vi "OUTPUT_DATA_PACKING_TYPE - Type.vi"(8 "error in (no error)":errorcluster) -> (0 "error out":errorcluster, 3 "OUTPUT_DATA_PACKING_TYPE_VALUE":i32)   [LabVIEW 2013]
doc: "<b>Buffer policy settings can be only unsafe in xiAPI LabVIEW library</b>\nUNSAFE : User gets pointer to internally allocated circle buffer and data may be overwritten by device.\nSAFE : Data from device will be copied to user allocated buffer or xiApi allocated memory."
uses:
  OUTPUT_DATA_PACKING_TYPE.ctl
  C:/Projects/Cameras3.x/xiLib/xiLIB_64bit/xiLIB/xiCamLib/API/x64/xiApi.NETX64.dll
  xiLIB_64bit/xiLIB/xiCamLib/API/x64/xiApi.NETX64.dll
panel:
  in  "OUTPUT_DATA_PACKING_TYPE":T1
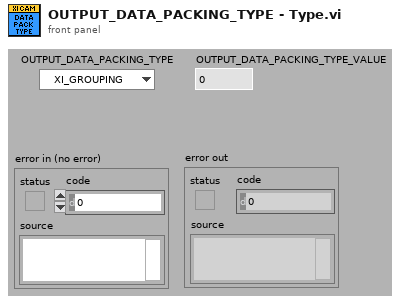
[diagram p1: front panel]
types:
  T1 = typedef "OUTPUT_DATA_PACKING_TYPE.ctl" = enum16{"XI_GROUPING", "PFNC_LSB_PACKING"}
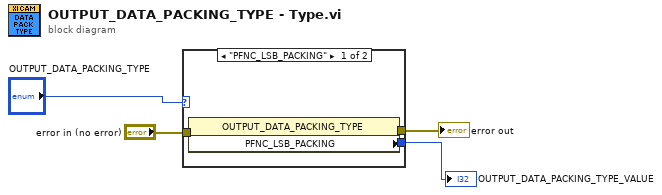
[diagram p0: block diagram]
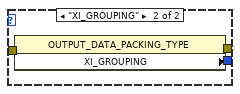
[diagram p2: hidden frame]
diagram:
  n1 = case shown="\"PFNC_LSB_PACKING\"" "OUTPUT_DATA_PACKING_TYPE" {
    tunnel: "error in (no error)" -> [w7 w10]
    tunnel: [w6 w9] -> w3
    tunnel: [w5 w8] -> w2
    frame "PFNC_LSB_PACKING" {
      n2 = property class="OUTPUT_DATA_PACKING_TYPE"(error in=w7) -> (error out=w6:errorcluster, "PFNC_LSB_PACKING"=w5:i32)  [unwired: 1 in, 1 out]
    }
    frame "XI_GROUPING" {
      n3 = property class="OUTPUT_DATA_PACKING_TYPE"(error in=w10) -> (error out=w9:errorcluster, "XI_GROUPING"=w8:i32)  [unwired: 1 in, 1 out]
    }
  }
  "error out" <- w3
  "OUTPUT_DATA_PACKING_TYPE_VALUE" <- w2
